vi "office_test.vi"() -> ()   [LabVIEW 2019]
panel:
  in  "Slide":dbl(slide) scale=0.0..100.0
  out "ip":string
  in  "stop":bool
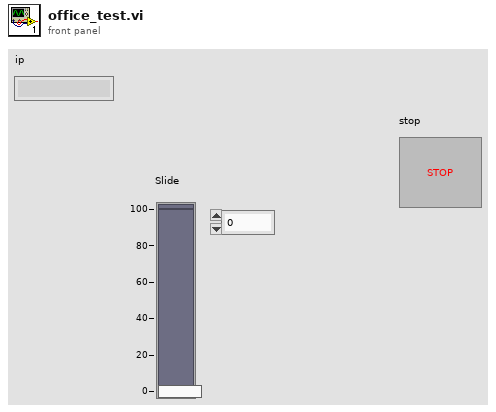
[diagram p1: front panel]
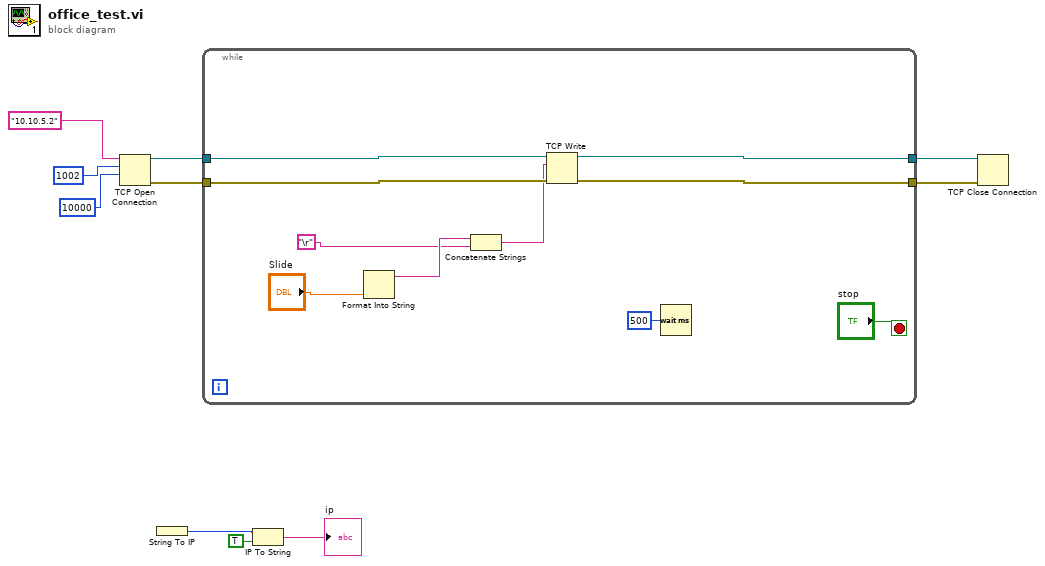
[diagram p0: block diagram]
diagram:
  n1 = TCP Open Connection(address="10.10.5.2", remote port or service name=u16 1002, timeout ms (60000)=10000) -> (connection ID=w7:refnum<k5>, error out=w6:errorcluster)  [unwired: 2 in]
  n2 = String To IP() -> (0:w10:u32)  [unwired: 1 in]
  n3 = while {
    tunnel: w7 -> [w19]
    tunnel: w6 -> [w18]
    tunnel: [w17] -> w5
    tunnel: [w16] -> w4
    stop <- "stop" stop-if-true
    n4 = Format Into String("Slide") -> (resulting string=w15:string)  [unwired: 3 in, 1 out]
    n5 = Concatenate Strings(w15, "\r") -> (w12:string)
    n6 = TCP Write(connection ID=w19, data in=w12, error in (no error)=w18) -> (connection ID out=w17:refnum<k5>, error out=w16:errorcluster)  [unwired: 1 in, 1 out]
    n7 = Wait (ms)(milliseconds to wait=u32 500) -> ()  [unwired: 1 out]
  }
  n8 = IP To String(1:TRUE ("dot notation? (F)"), 2:w10) -> (0:→"ip":string)
  n9 = TCP Close Connection(connection ID=w5, error in (no error)=w4) -> ()  [unwired: 1 in, 2 out]
